vi "Format.vi"(8 "error in (no error)":errorcluster, 10 "log record":T1 {"timestamp" format="%<%x %.3X>T"}, 11 "Format String in":refnum<class "Format String.lvclass">) -> (0 "error out":errorcluster, 2 "log line":string, 3 "Format String out":refnum<class "Format String.lvclass">)   [LabVIEW 2018, in "GLog.lvlib" / "Format String.lvclass"]
uses:
  Format String.lvclass
  Log Record.ctl
  logger_class/Internal Log Levels.ctl
  Format String.lvclass/Format String.ctl
  GLog.lvlib
panel:
  # "Connector Pane"
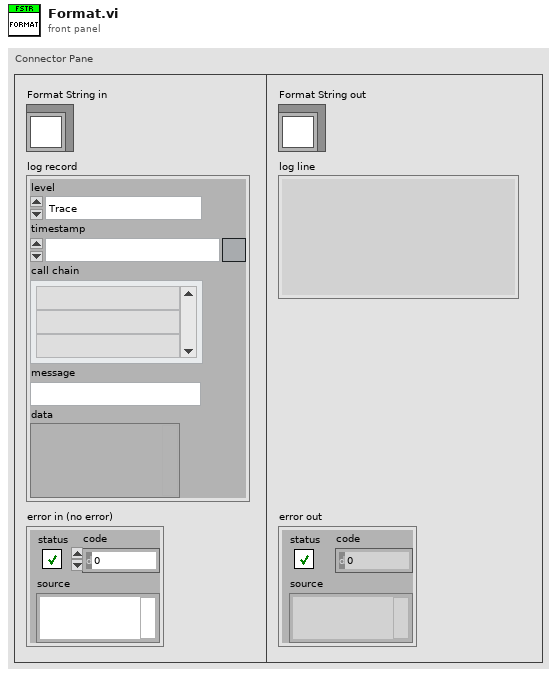
[diagram p1: front panel]
types:
  T1 = typedef "GLog.lvlib/Log Record.ctl" = cluster{"level":T2, "timestamp":timestamp, "call chain":string[], "message":string, "data":variant}
  T2 = typedef "GLog.lvlib/Internal Log Levels.ctl" = enum16{"Trace", "Debug", "Info", "Warning", "Error", "Critical", "Internal"}
  T3 = typedef "GLog.lvlib/Format String.lvclass/Call Chain Format Parameters.ctl" = cluster{"Delimiter":string, "# of Callers":i32, "Remove Namespaces?":bool, "String Length":i32}
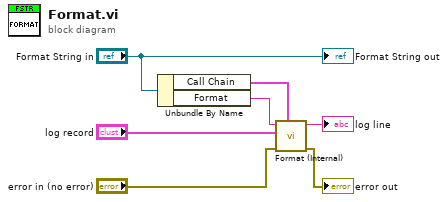
[diagram p0: block diagram]
diagram:
  n1 = Unbundle By Name("Format String in") -> ("Call Chain"=w3:T3, "Format"=w7:string)
  n2 = call "Format (Internal).vi"("call chain format params"=w3, "error in (no error)"="error in (no error)", "log record"="log record", "format string"=w7) -> ("error out"=→"error out":errorcluster, "formatted string"=→"log line":string)  [unwired: 6 in]
  "Format String out" <- "Format String in"
